vi "Configure OVP.vi"(8 "error in (no error)":errorcluster, 9 "Enable OVP (T: Enable)":bool=TRUE, 10 "Voltage Limit (66.000 V)":dbl=66.0 min=0.0 max=156.0 step=0.001 format="%.3g", 11 "VISA resource name":refnum<visa-resource-name>) -> (0 "error out":errorcluster, 3 "VISA resource name out":refnum<visa-resource-name>)   [LabVIEW 2021, in "BK Precision 9200 Series.lvlib"]
doc: "Configures over voltage protection (OVP) of the power supply."
uses:
  <instrlib>/BK Precision 9200 Series/BK Precision 9200 Series.lvlib
panel:
  # "V"
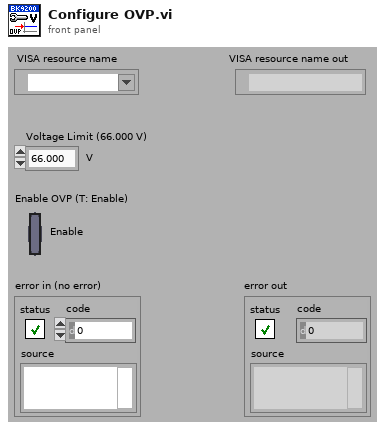
[diagram p1: front panel]
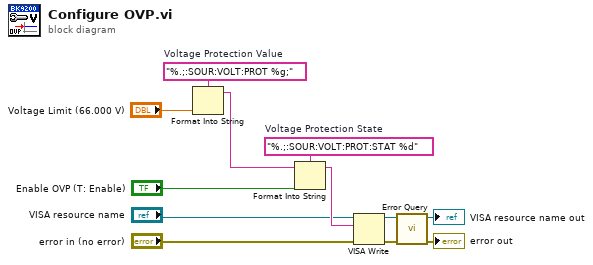
[diagram p0: block diagram]
diagram:
  w9 = "%.;:SOUR:VOLT:PROT:STAT %d"  # Voltage Protection State
  w10 = "%.;:SOUR:VOLT:PROT %g;"  # Voltage Protection Value
  n1 = Format Into String(format string=w10, "Voltage Limit (66.000 V)") -> (resulting string=w1:string)  [unwired: 2 in, 1 out]
  n2 = Format Into String(format string=w9, initial string=w1, "Enable OVP (T: Enable)") -> (resulting string=w8:string)  [unwired: 1 in, 1 out]
  n3 = VISA Write(VISA resource name="VISA resource name", write buffer=w8, error in (no error)="error in (no error)") -> (VISA resource name out=w6:refnum<visa-resource-name>, error out=w5:errorcluster)  [unwired: 1 out]
  n4 = call <instrlib>:"Error Query.vi"("error in (no error)"=w5, "VISA resource name"=w6) -> ("error out"=→"error out":errorcluster, "VISA resource name out"=→"VISA resource name out":refnum<visa-resource-name>)  [unwired: 6 in, 2 out]
